vi "Define Level Keys.vi"(8 "error in":errorcluster, 9 "Level Down Keys":string[](array[string]), 10 "Level Up Keys":string[](array[string]), 11 "Fast Tree in":refnum<class "Fast Tree.lvclass">) -> (0 "error out":errorcluster, 3 "Fast Tree out":refnum<class "Fast Tree.lvclass">)   [LabVIEW 2019, in "Fast Tree.lvclass"]
uses:
  Fast Tree.lvclass
  Fast Tree.lvclass/Fast Tree.ctl
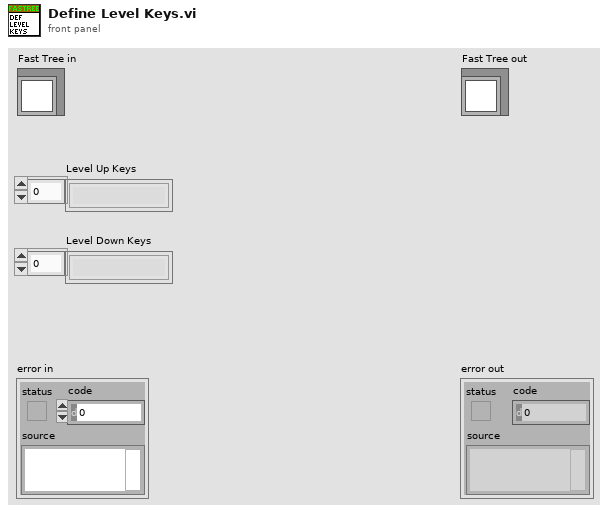
[diagram p1: front panel]
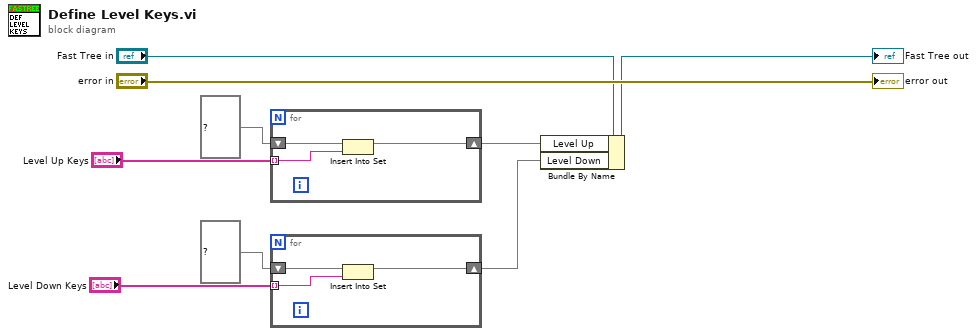
[diagram p0: block diagram]
diagram:
  n1 = for {
    shift-right: [w11] -> w4
    shift-left: set{string} {} ("set") -> [w12]
    tunnel: "Level Up Keys" -> [w10] mode=indexing
    n2 = Insert Into Set(10:w10, 11:w12) -> (3:w11:set{string})  [unwired: 1 out]
  }
  n3 = for {
    shift-right: [w14] -> w3
    shift-left: set{string} {} ("set") -> [w15]
    tunnel: "Level Down Keys" -> [w13] mode=indexing
    n4 = Insert Into Set(10:w13, 11:w15) -> (3:w14:set{string})  [unwired: 1 out]
  }
  n5 = Bundle By Name(cluster="Fast Tree in", "Level Up"=w4, "Level Down"=w3) -> (→"Fast Tree out":refnum<class "Fast Tree.lvclass">)
  "error out" <- "error in"
